vi "GET_publisher_by_id.vi"(8 "error in (no error)":errorcluster, 10 "publisher id":i32, 11 "REST Client in":refnum<class "REST Client.lvclass">) -> (0 "error out":errorcluster, 1 "good get":bool, 2 "local volume":T1, 3 "REST Client out":refnum<class "REST Client.lvclass">, 4 "Status Code":u16)   [LabVIEW 2024, in "CV_RESTful_Lib.lvlib"]
uses:
  CV_RESTful_Lib.lvlib
  <vilib>/addons/_JKI.lib/REST Client/classes/REST Client/REST Client.lvclass
  typedefs/local_publisher--cluster.ctl
  <vilib>/addons/_JKI.lib/REST Client/classes/REST Client/HTTP Header.ctl
  <vilib>/NI/Advanced HTTP Client/Header--Combo Box.ctl
  typedefs/cv_publisher--cluster.ctl
  typedefs/cv_publisher.results--cluster.ctl
  typedefs/cv_volume.issue--cluster.ctl
  <vilib>/NI/Advanced HTTP Client/Session.lvclass
  <userlib>/_OpenG.lib/string/string.llb/openg_string.lvlib
  <vilib>/addons/_JKI.lib/Serialization/JSON/JKI JSON Serialization.lvlib
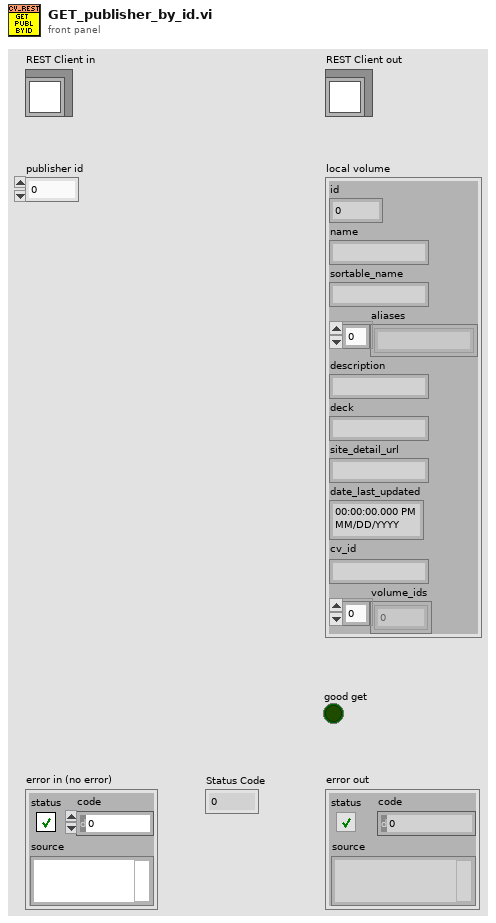
[diagram p1: front panel]
types:
  T1 = typedef "CV_RESTful_Lib.lvlib/local_publisher--cluster.ctl" = cluster{"id":i32, "name":string, "sortable_name":string, "aliases":string[], "description":string, "deck":string, "site_detail_url":string, "date_last_updated":timestamp, "cv_id":string, "volume_ids":i32[]}
  T2 = typedef "REST Client.lvlib/REST Client.lvclass/HTTP Header.ctl" = cluster{"header":T3, "value":string}
  T3 = typedef "lib_NI_Advanced HTTP Client.lvlib/Session.lvclass/Header--Combo Box.ctl" = string
  T4 = typedef "CV_RESTful_Lib.lvlib/cv_publisher--cluster.ctl" = cluster{"error":string, "limit":i32, "offset":i32, "number_of_page_results":i32, "number_of_total_results":i32, "status_code":i32, "results":T5}
  T5 = typedef "CV_RESTful_Lib.lvlib/cv_publisher.results--cluster.ctl" = cluster{"aliases":string, "date_last_updated":timestamp, "deck":string, "description":string, "id":i32, "name":string, "site_detail_url":string, "volumes":T6[]}
  T6 = typedef "CV_RESTful_Lib.lvlib/cv_volume.issue--cluster.ctl" = cluster{"id":i32}
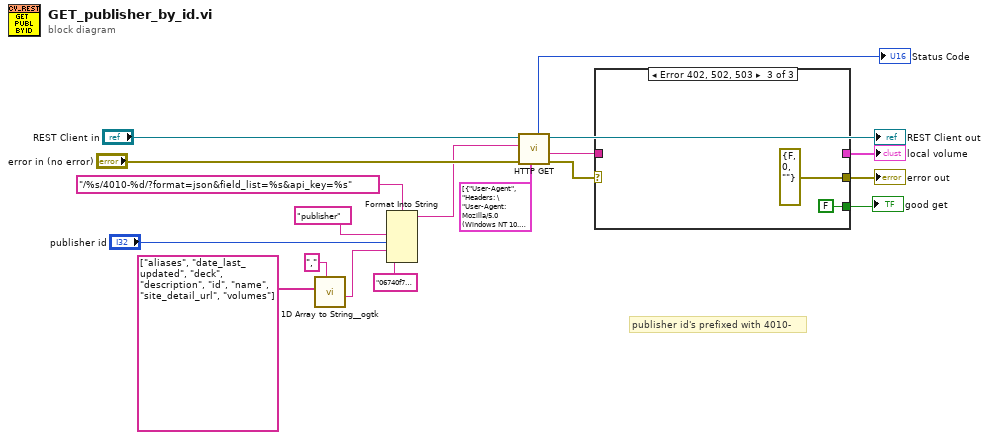
[diagram p0: block diagram]
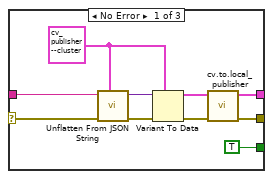
[diagram p2: hidden frame]
diagram:
  # "publisher id's prefixed with 4010-"
  n1 = call <userlib>:"1D Array to String__ogtk.vi"("delimiter (Tab)"=",", "Array of Strings"=string[] ["aliases", "date_last_updated", "deck", "description", "id", "name", "site_detail_url", "volumes"]) -> ("delimited string"=w9:string)  [unwired: 9 in]
  n2 = Format Into String(format string="/%s/4010-%d/?format=json&field_list=%s&api_key=%s", "publisher" ("resource"), "publisher id", w9, "06740f73403e0b211d597c50ea94c7f16ea5e8ea") -> (resulting string=w14:string)  [unwired: 2 in, 1 out]
  n3 = call-dynamic "HTTP GET.vi"("request specific headers"=T2[] [{"header"="User-Agent", "value"="Headers: \"User-Agent: Mozilla/5.0 (Windows NT 10.0; Win64; x64) AppleWebKit/537.36 (KHTML, like Gecko) Chrome/91.0.4472.101 Safari/537.36\""}], "error in (no error)"="error in (no error)", "Path"=w14, "REST Client in"="REST Client in") -> ("error out"=w2:errorcluster, "Response body"=w8:string, "REST Client out"=→"REST Client out":refnum<class "REST Client.lvclass">, "Status Code"=→"Status Code":u16)  [unwired: 2 in, 2 out]
  n4 = case shown="Error 402, 502, 503" w2 {
    selector: w2 -> [w20 w29 _]
    tunnel: w8 -> [w28 _ _]
    tunnel: [w23 _ _] -> w5
    tunnel: [w21 w29 errorcluster {"status"=FALSE, "code"=0, "source"=""} ("error in (no error)")] -> w4
    tunnel: [TRUE _ FALSE] -> w1
    frame No Error {
      w26 = T4 {"error"="", "limit"=0, "offset"=0, "number_of_page_results"=0, "number_of_total_results"=0, "status_code"=0, "results"={"aliases"="", "date_last_updated"=timestamp(0 s since 1904-01-01), "deck"="", "description"="", "id"=0, "name"="", "site_detail_url"="", "volumes"=[]}} ("volume")
      n5 = call <vilib>:"Unflatten From JSON String.vi"("Type and Defaults"=w26, "error in"=w20, "JSON String"=w28) -> ("error out"=w25:errorcluster, "Variant"=w27:variant)  [unwired: 7 in]
      n6 = Variant To Data(error in=w25, type=w26, Variant=w27) -> (data=w24:T4, error out=w22:errorcluster)
      n7 = call "cv.to.local_publisher.vi"("error in (no error)"=w22, "cv publisher"=w24) -> ("error out"=w21:errorcluster, "local publisher"=w23:T1)  [unwired: 8 in]
    }
    frame Default {
    }
    frame Error {
    }
  }
  "error out" <- w4
  "local volume" <- w5
  "good get" <- w1
